vi "TwCloseH5.vi"(1 "filename":string, 2 "error in (no error)":errorcluster) -> (0 "error out":errorcluster)   [LabVIEW 2009]
uses:
  TwH5Dll.dll
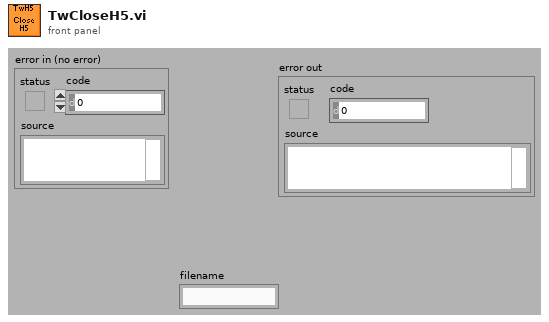
[diagram p1: front panel]
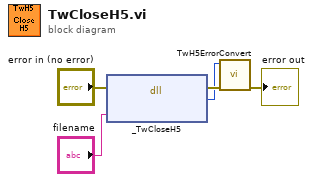
[diagram p0: block diagram]
diagram:
  n1 = dll-call lib="C:/src/85_TofDaq_current/DllWrappers/LabView/TwH5Dll/TwH5Dll.dll" fn="_TwCloseH5"(error in="error in (no error)", "filename"="filename") -> (error out=w4:errorcluster, "TwRetVal"=w3:i32)  [unwired: 3 in, 1 out]
  n2 = call "TwH5ErrorConvert.vi"("error in (no error)"=w4, "error code"=w3) -> ("error out"=→"error out":errorcluster)  [unwired: 9 out]
